vi "Write Image.vi"(8 "error in (no error)":errorcluster, 9 "2D Picture":picture, 11 "I2C OLED in":refnum<class "OLED.lvclass">) -> (0 "error out":errorcluster, 3 "I2C OLED out":refnum<class "OLED.lvclass">)   [LabVIEW 2020, in "CTI-Peripheral.lvlib" / "OLED.lvclass"]
uses:
  OLED.lvclass
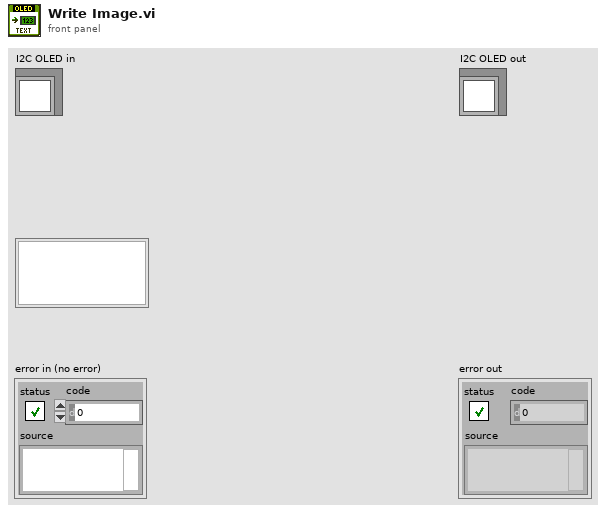
[diagram p1: front panel]
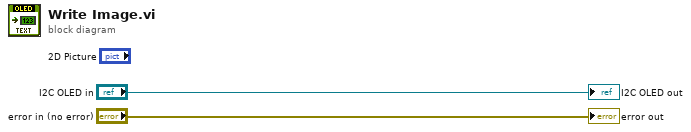
[diagram p0: block diagram]
diagram:
  "error out" <- "error in (no error)"
  "I2C OLED out" <- "I2C OLED in"
